vi "_Test_EBD_Generator.vi"() -> ()   [LabVIEW 2020]
panel:
  in  "file path (use dialog)":path
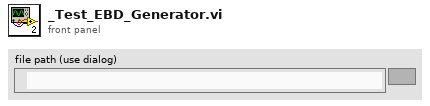
[diagram p1: front panel]
types:
  T1 = enum16{"open", "replace", "create", "open or create", "replace or create", "replace or create with confirmation"}
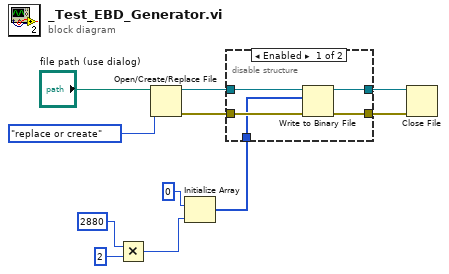
[diagram p0: block diagram]
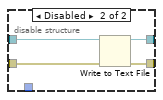
[diagram p2: hidden frame]
diagram:
  n1 = Multiply(x=2880 ("dimension size"), y=2) -> (x*y=w3:i32)
  n2 = Open/Create/Replace File(file path (use dialog)="file path (use dialog)", operation (0:open)=T1."replace or create") -> (refnum out=w11:refnum<file>, error out=w10:errorcluster)  [unwired: 4 in, 1 out]
  n3 = Initialize Array(u8 0, w3) -> (w2:u8[])
  n4 = disable-structure shown="Enabled" {
    disable-tunnel: w11 -> [w16 w19]
    disable-tunnel: w10 -> [w15 w18]
    disable-tunnel: [w14 w17] -> w9
    disable-tunnel: [w13 w20] -> w8
    disable-tunnel: w2 -> [w12 _]
    frame Enabled {
      n5 = Write to Binary File(file (use dialog)=w16, data=w12, error in=w15) -> (refnum out=w14:refnum<file>, error out=w13:errorcluster)  [unwired: 3 in, 1 out]
    }
    frame Disabled {
      n6 = Write to Text File(file (use dialog)=w19, error in=w18) -> (refnum out=w17:refnum<file>, error out=w20:errorcluster)  [unwired: 2 in, 1 out]
    }
  }
  n7 = Close File(refnum=w9, error in=w8) -> ()  [unwired: 2 out]
